vi "Merge Assertion Status.vi"(10 "New":T1, 11 "Current":T1) -> (1 "Changed?":bool, 3 "Merged":T1)   [LabVIEW 2020, in "Result.lvlib"]
uses:
  Result.lvlib
  Status.ctl
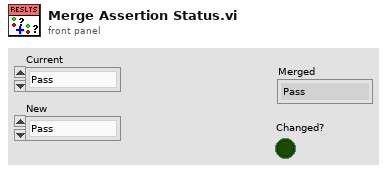
[diagram p1: front panel]
types:
  T1 = typedef "Result.lvlib/Status.ctl" = enum16{"Pass", "Fail", "Error", "Skipped", "Setup Error", "Broken", "Teardown Error"}
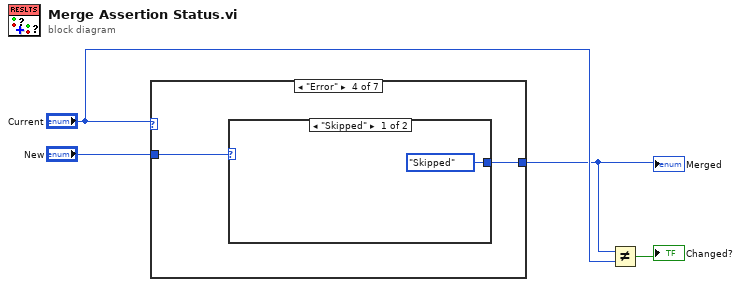
[diagram p0: block diagram]
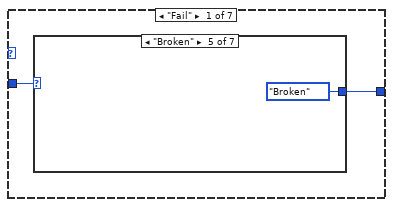
[diagram p2: hidden frame]
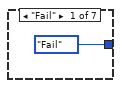
[diagram p3: hidden frame]
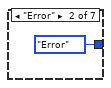
[diagram p4: hidden frame]
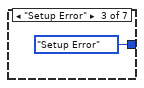
[diagram p5: hidden frame]
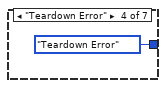
[diagram p6: hidden frame]
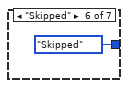
[diagram p7: hidden frame]
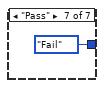
[diagram p8: hidden frame]
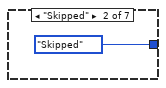
[diagram p9: hidden frame]
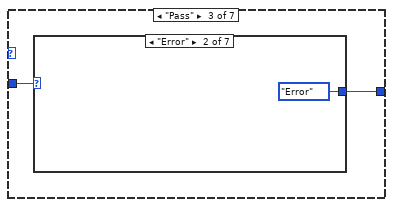
[diagram p10: hidden frame]
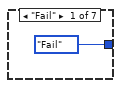
[diagram p11: hidden frame]
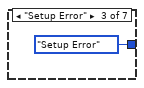
[diagram p12: hidden frame]
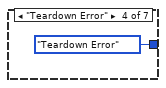
[diagram p13: hidden frame]
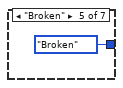
[diagram p14: hidden frame]
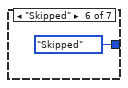
[diagram p15: hidden frame]
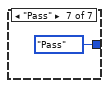
[diagram p16: hidden frame]
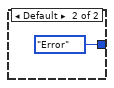
[diagram p17: hidden frame]
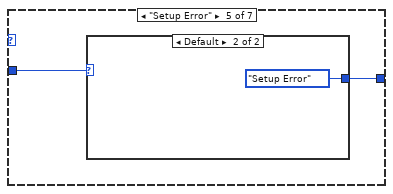
[diagram p18: hidden frame]
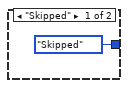
[diagram p19: hidden frame]
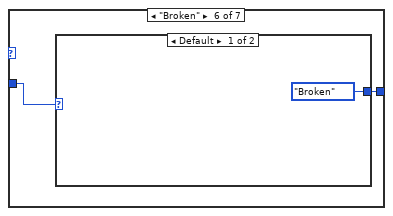
[diagram p20: hidden frame]
diagram:
  n1 = case shown="\"Error\"" "Current" {
    tunnel: "New" -> [w6 _ w16 w24 w28 w32 w36]
    tunnel: [w5 Status."Skipped" ("Merged Status") w15 w25 w29 w33 w37] -> w2
    frame "Fail" {
      n2 = case shown="\"Broken\"" w6 {
        tunnel: [Status."Fail" ("Merged Status") Status."Error" ("Merged Status") Status."Setup Error" ("Merged Status") Status."Teardown Error" ("Merged Status") Status."Broken" ("Merged Status") Status."Skipped" ("Merged Status") Status."Fail" ("Merged Status")] -> w5
        frame "Fail" {
        }
        frame "Error" {
        }
        frame "Setup Error" {
        }
        frame "Teardown Error" {
        }
        frame "Broken" {
        }
        frame "Skipped" {
        }
        frame "Pass" {
        }
      }
    }
    frame "Skipped" {
    }
    frame "Pass" {
      n3 = case shown="\"Error\"" w16 {
        tunnel: [Status."Fail" ("Merged Status") Status."Error" ("Merged Status") Status."Setup Error" ("Merged Status") Status."Teardown Error" ("Merged Status") Status."Broken" ("Merged Status") Status."Skipped" ("Merged Status") Status."Pass" ("Merged Status")] -> w15
        frame "Fail" {
        }
        frame "Error" {
        }
        frame "Setup Error" {
        }
        frame "Teardown Error" {
        }
        frame "Broken" {
        }
        frame "Skipped" {
        }
        frame "Pass" {
        }
      }
    }
    frame "Error" {
      n4 = case shown="\"Skipped\"" w24 {
        tunnel: [Status."Skipped" ("Merged Status") Status."Error" ("Merged Status")] -> w25
        frame "Skipped" {
        }
        frame Default {
        }
      }
    }
    frame "Setup Error" {
      n5 = case shown="Default" w28 {
        tunnel: [Status."Skipped" ("Merged Status") Status."Setup Error" ("Merged Status")] -> w29
        frame "Skipped" {
        }
        frame Default {
        }
      }
    }
    frame "Broken" {
      n6 = case shown="Default" w32 {
        tunnel: [Status."Broken" ("Merged Status") Status."Setup Error" ("Merged Status")] -> w33
        frame Default {
        }
        frame "Setup Error" {
        }
      }
    }
    frame "Teardown Error" {
      n7 = case shown="Default" w36 {
        tunnel: [Status."Skipped" ("Merged Status") Status."Teardown Error" ("Merged Status")] -> w37
        frame "Skipped" {
        }
        frame Default {
        }
      }
    }
  }
  "Merged" <- w2
  n8 = Not Equal?(x=w2, y="Current") -> (x != y?=→"Changed?":bool)
